vi "Check String Comparison.vi"(8 "error in (no error)":errorcluster, 10 "Expected String":string, 11 "String":string) -> (0 "error out":errorcluster, 2 "Found?":bool, 3 "string out":string)   [LabVIEW 2019, in "Instrument Addon Engine.lvlib"]
uses:
  Instrument Addon Engine.lvlib
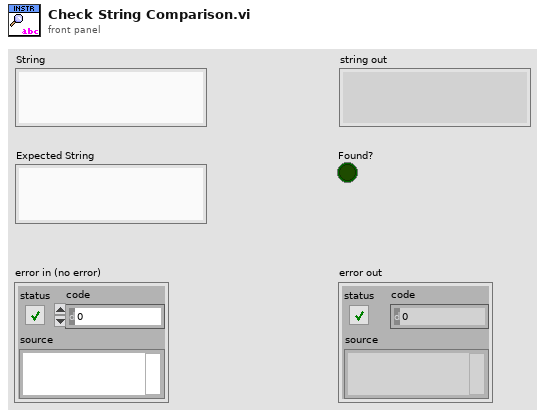
[diagram p1: front panel]
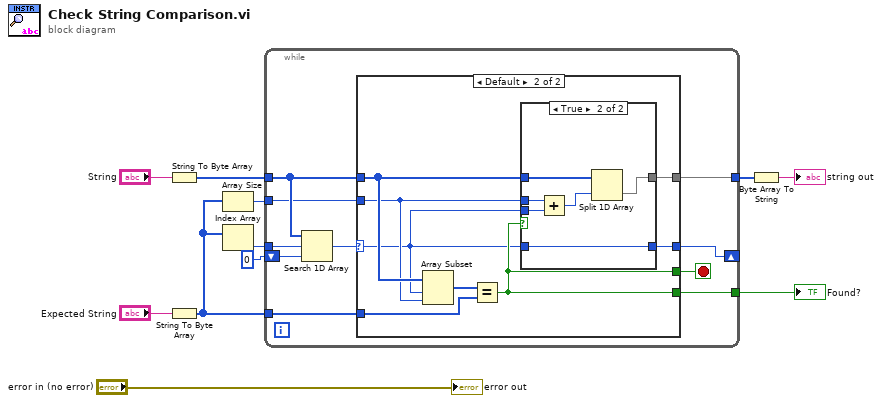
[diagram p0: block diagram]
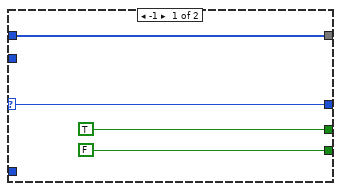
[diagram p2: hidden frame]
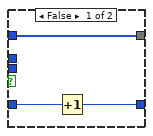
[diagram p3: hidden frame]
diagram:
  n1 = String To Byte Array(string="String") -> (unsigned byte array=w9:u8[])
  n2 = String To Byte Array(string="Expected String") -> (unsigned byte array=w6:u8[])
  n3 = Array Size(array=w6) -> (size(s)=w8:i32)
  n4 = Index Array(array=w6) -> (element=w5:u8)  [unwired: 1 in]
  n5 = while {
    tunnel: w9 -> [w20]
    tunnel: w6 -> [w18]
    tunnel: w8 -> [w19]
    tunnel: [w16] -> w7
    tunnel: w5 -> [w15]
    tunnel: [w14] -> w3
    shift-right: [w12] -> _
    shift-left: 0 ("index of element") -> [w13]
    stop <- w17 stop-if-true
    n6 = Search 1D Array(1D array=w20, element=w15, start index (0)=w13) -> (index of element=w21:i32)
    n7 = case shown="Default" w21 {
      selector: w21 -> [w22 w26]
      tunnel: w20 -> [w23 w30]
      tunnel: w19 -> [_ w29]
      tunnel: w18 -> [_ w33]
      tunnel: [TRUE w31] -> w17
      tunnel: [FALSE w31] -> w16
      tunnel: [w23 w28] -> w14
      tunnel: [w22 w27] -> w12
      frame -1 {
      }
      frame Default {
        n8 = Array Subset(array=w30, index=w26, length=w29) -> (w32:u8[])
        n9 = Equal?(x=w32, y=w33) -> (x = y?=w31:bool)
        n10 = case shown="True" w31 {
          tunnel: w30 -> [w36 w40]
          tunnel: w26 -> [_ w42]
          tunnel: w29 -> [_ w41]
          tunnel: [w36 w38] -> w28
          tunnel: [w34 w37] -> w27
          tunnel: w26 -> [w35 w37]
          frame False {
            n11 = Increment(x=w35) -> (x+1=w34:i32)
          }
          frame True {
            n12 = Add(x=w41, y=w42) -> (x+y=w39:i32)
            n13 = Split 1D Array(array=w40, index=w39) -> (second subarray=w38:u8[])  [unwired: 1 out]
          }
        }
      }
    }
  }
  "Found?" <- w7
  n14 = Byte Array To String(unsigned byte array=w3) -> (string=→"string out":string)
  "error out" <- "error in (no error)"
